vi "Path2LineArray.vi"(11 "Path":T3) -> (3 "LineArray":T1=[{"X"=0.0, "Y"=0.0, "OnOff"=TRUE}, {"X"=0.0, "Y"=0.5, "OnOff"=TRUE}, {"X"=0.5, "Y"=1.0, "OnOff"=TRUE}, {"X"=1.0, "Y"=0.5, "OnOff"=TRUE}, {"X"=0.5, "Y"=0.0, "OnOff"=TRUE}, {"X"=0.0, "Y"=0.5, "OnOff"=TRUE}, {"X"=0.0, "Y"=0.0, "OnOff"=TRUE}])   [LabVIEW 2014]
uses:
  TypeDefs/Point2DwSlope.ctl
  TypeDefs/XYonOffArray.ctl
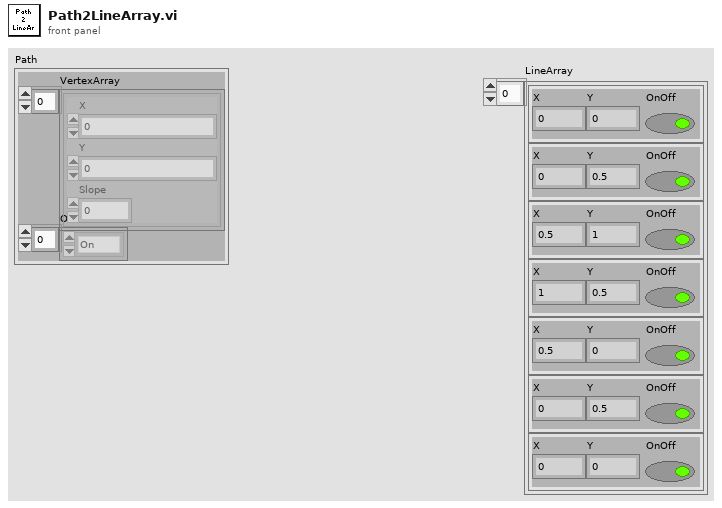
[diagram p1: front panel]
types:
  T1 = typedef "XYonOffArray.ctl" = cluster{"X":dbl, "Y":dbl, "OnOff":bool}[]
  T2 = typedef "Point2DwSlope.ctl" = cluster{"X":sgl, "Y":sgl, "Slope":dbl}
  T3 = cluster{"VertexArray":T2[], "OnOffAr":enum16{"On", "Off"}[]}
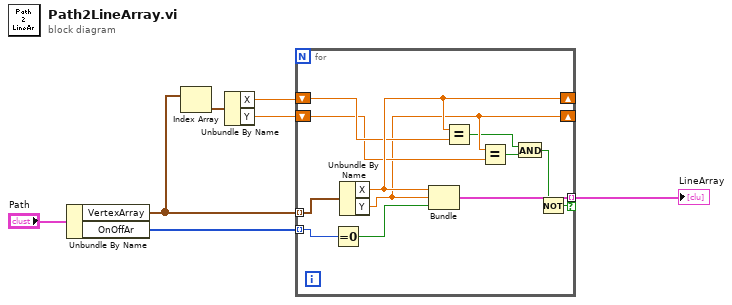
[diagram p0: block diagram]
diagram:
  n1 = Unbundle By Name("Path") -> ("VertexArray"=w4:T2[], "OnOffAr"=w6:enum16{"On", "Off"}[])
  n2 = Index Array(array=w4) -> (element=w3:T2)  [unwired: 1 in]
  n3 = Unbundle By Name(w3) -> ("X"=w2:sgl, "Y"=w1:sgl)
  n4 = for {
    tunnel: w4 -> [w19] mode=indexing
    tunnel: w6 -> [w18] mode=indexing
    tunnel: [w16] -> w5 mode=indexing if=w9
    shift-right: [w12] -> _
    shift-left: w1 -> [w13]
    shift-right: [w15] -> _
    shift-left: w2 -> [w14]
    n5 = Equal To 0?(x=w18) -> (x = 0?=w17:bool)
    n6 = Unbundle By Name(w19) -> ("X"=w15:sgl, "Y"=w12:sgl)
    n7 = Bundle("X"=w15, "Y"=w12, w17) -> (w16:cluster{"X":sgl, "Y":sgl, bool})  [unwired: 1 in]
    n8 = Equal?(x=w15, y=w14) -> (x = y?=w10:bool)
    n9 = Equal?(x=w12, y=w13) -> (x = y?=w11:bool)
    n10 = And(x=w10, y=w11) -> (x .and. y?=w8:bool)
    n11 = Not(x=w8) -> (.not. x?=w9:bool)
  }
  "LineArray" <- w5
